vi "0002H_水中油_监测值&信号值读取.vi"(8 "error in (no error)":errorcluster caption="错误输入（无错误）", 11 "MB_Serial session in":refnum<class "MB_Master_Serial.lvclass">) -> (0 "error out":errorcluster caption="错误输出", 2 "浊度":T1, 3 "MB_Serial session out":refnum<class "MB_Master_Serial.lvclass">)   [LabVIEW 2016, in "斯坦道多参数.lvlib"]
uses:
  <vilib>/Plasmionique/MB Master/MB Master.lvlib
  <vilib>/Plasmionique/MB Master/MB_Master_Serial/MB_Master_Serial.lvclass
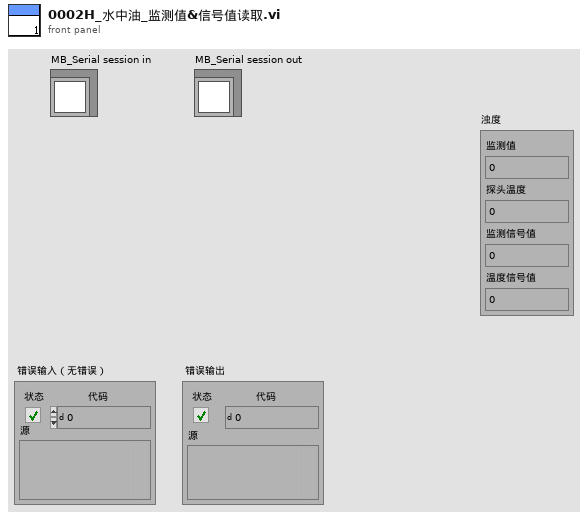
[diagram p1: front panel]
types:
  T1 = cluster{"监测值":dbl, "探头温度":dbl, "监测信号值":dbl, "温度信号值":dbl}
  T2 = cluster{"数组 2[0]":sgl, "数组 2[1]":sgl, "数组 2[2]":sgl, "数组 2[3]":sgl}
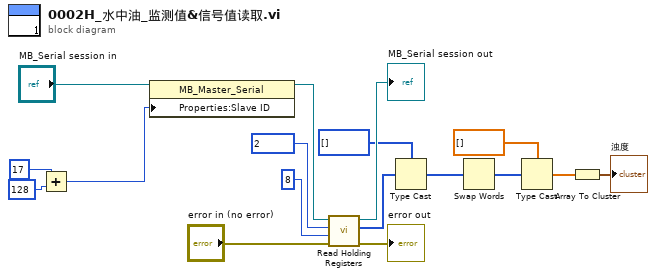
[diagram p0: block diagram]
diagram:
  n1 = Add(x=u16 17, y=u16 128) -> (x+y=w1:u16)
  n2 = property class="MB_Master_Serial"(reference="MB_Serial session in", "Properties:Slave ID"=w1) -> (reference out=w4:refnum<class "MB_Master_Serial.lvclass">)  [unwired: 1 in, 1 out]
  n3 = call <vilib>:"Read Holding Registers.vi"("error in (no error)"="error in (no error)", "quantity"=u16 8, "starting address"=u16 2, "MB session in"=w4) -> ("error out"=→"error out":errorcluster, "Registers"=w7:u16[], "MB session out"=→"MB_Serial session out":refnum<class "MB_Master_Serial.lvclass">)  [unwired: 5 in]
  n4 = Type Cast(type=u32[] [] ("数组 2"), x=w7) -> (*(type *) &x=w8:u32[])
  n5 = Swap Words(1:w8) -> (0:w6:u32[])
  n6 = Type Cast(type=sgl[] [] ("数组 2"), x=w6) -> (*(type *) &x=w11:sgl[])
  n7 = Array To Cluster(array=w11) -> (cluster=→"浊度":T2)
